vi "Get Delay.vi"(8 "error in (no error)":errorcluster, 11 "Instrument.Delay in":refnum<class "Instrument.Aerotech.lvclass">) -> (0 "error out":errorcluster, 2 "Delay (ps)":dbl, 3 "Instrument.Delay out":refnum<class "Instrument.Aerotech.lvclass">, 4 "Finished?":bool)   [LabVIEW 2016, in "Instrument.Aerotech.lvclass"]
uses:
  Instrument.Aerotech.lvclass
  Aerotech-Ensemble-LabVIEW/8.2/Motion/EnableSingle.vi
  Aerotech-Ensemble-LabVIEW/8.2/Motion/DisableSingle.vi
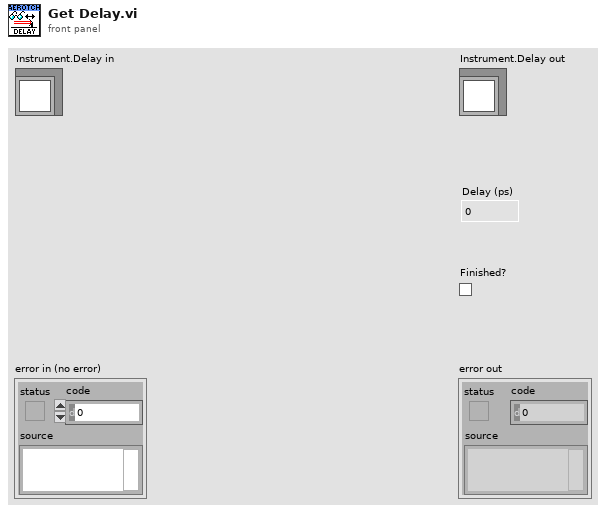
[diagram p1: front panel]
types:
  T1 = typedef "ControllerDiagPacket.ctl" = cluster{"Count":i32, "Packet Time":i64, "Axes":T2[], "error":errorcluster}
  T2 = typedef "AxisDiagPacket.ctl" = cluster{"Axis Name":string, "Acceleration Command":dbl, "Amplifier Temperature":sgl, "Analog Input 0":dbl, "Analog Input 1":dbl, "Analog Output 0":dbl, "Analog Output 1":dbl, "Axis Fault (num)":i32, "Axis Fault (str)":string, "Axis Fault (bits)":cluster{"AmplifierFault":bool, "AmplifierTemperatureFault":bool, "CcwEndOfTravelLimitFault":bool, "CcwSoftwareLimitFault":bool, "CommunicationLostFault":bool, "CwEndOfTravelLimitFault":bool, "CwSoftwareLimitFault":bool, "EmergencyStopFault":bool, "EncoderFault":bool, "ExternalFault":bool, "FeedbackScalingFault":bool, "HallSensorFault":bool, "MarkerSearchFault":bool, "MaxVelocityCommandFault":bool, "MotorTemperatureFault":bool, "None":bool, "OverCurrentFault":bool, "PositionErrorFault":bool, "PositionFeedbackFault":bool, "VelocityErrorFault":bool, "VelocityFeedbackFault":bool, "VoltageClampFault":bool}, "Axis Status (num)":i32, "Axis Status (str)":string, "Axis Status (bits)":cluster{"AccelerationPhase":bool, "AutofocusActive":bool, "BrakeOutput":bool, "CalibrationActive":bool, "CalibrationEnabled":bool, "CcwEndOfTravelLimitInput":bool, "CommandShapingFilterDone":bool, "CosineEncoderError":bool, "CurrentClamp":bool, "CwEndOfTravelLimitInput":bool, "DecelerationPhase":bool, "EmergencyStopInput":bool, "Enabled":bool, "GantryMasterActive":bool, "GantryModeActive":bool, "HallAInput":bool, "HallBInput":bool, "HallCInput":bool, "Homed":bool, "HomeLimitInput":bool, "Homing":bool, "InPosition":bool, "InPosition2":bool, "JoystickControl":bool, "MarkerInput":bool, "MasterMotionSuppressed":bool, "MasterSlaveControl":bool, "MotionIsCw":bool, "MoveActive":bool, "None":bool, "PositionCaptureActive":bool, "ServoControl":bool, "SineEncoderError":bool}, "Current Command":sgl, "Current Error":sgl, "Current Feedback":sgl, "Digital Input 0":i32, "Digital Input 1":i32, "Digital Input 2":i32, "Digital Output 0":i32, "Digital Output 1":i32, "Digital Output 2":i32, "Position Feedback Auxiliary":dbl, "Position Command":dbl, "Position Error":dbl, "Position Feedback":dbl, "Program Position Command":dbl, "Program Position Error":dbl, "Program Position Feedback":dbl, "Velocity Command":dbl, "Velocity Error":dbl, "Velocity Feedback":dbl}
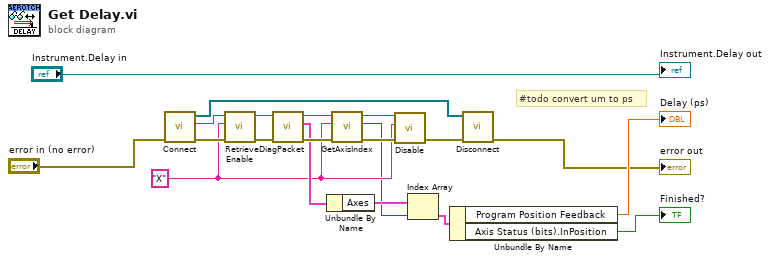
[diagram p0: block diagram]
diagram:
  w6 = "X" ("axis name")
  # "#todo convert um to ps"
  n1 = call "Connect.vi"("error in (no error)"="error in (no error)") -> ("error out"=w17:errorcluster, "controller"=w20:refnum<k24>, "controllers"=w19:refnum<k24>[])  [unwired: 8 in]
  n2 = call-poly "Enable.vi"("error in (no error)"=w17, "axis name"=w6, "controller in"=w20) -> ("error out"=w14:errorcluster, "controller out"=w13:refnum<k24>)  [unwired: 7 in]
  n3 = call "RetrieveDiagPacket.vi"("error in (no error)"=w14, "Controller In"=w13) -> ("error out"=w11:errorcluster, "ControllerDiagPacket"=w8:T1, "Controller Out"=w12:refnum<k24>)  [unwired: 7 in]
  n4 = Unbundle By Name(w8) -> ("Axes"=w7:T2[])
  n5 = call "GetAxisIndex.vi"("error in (no error)"=w11, "axis name"=w6, "controller in"=w12) -> ("error out"=w9:errorcluster, "axis index"=w5:i32, "controller out"=w10:refnum<k24>)  [unwired: 6 in]
  n6 = call-poly "Disable.vi"("error in (no error)"=w9, "axis name"=w6, "controller in"=w10) -> ("error out"=w18:errorcluster)  [unwired: 7 in, 1 out]
  n7 = Index Array(array=w7, index=w5) -> (element=w4:T2)
  n8 = Unbundle By Name(w4) -> ("Program Position Feedback"=→"Delay (ps)":dbl, "Axis Status (bits).InPosition"=→"Finished?":bool)
  n9 = call "Disconnect.vi"("error in (no error)"=w18, "controllers"=w19) -> ("error out"=→"error out":errorcluster)  [unwired: 9 in]
  "Instrument.Delay out" <- "Instrument.Delay in"
